vi "VI_PC.vi"() -> ()   [LabVIEW 2018]
uses:
  <vilib>/Utility/inputDevices.llb/joystickAcquire.vi
  <vilib>/Utility/inputDevices.llb/closeJoystick.vi
panel:
  out "direction info":T1
  out "button info":T2
  out "axis info":T3
  in  "stop":bool
  out "error out":errorcluster
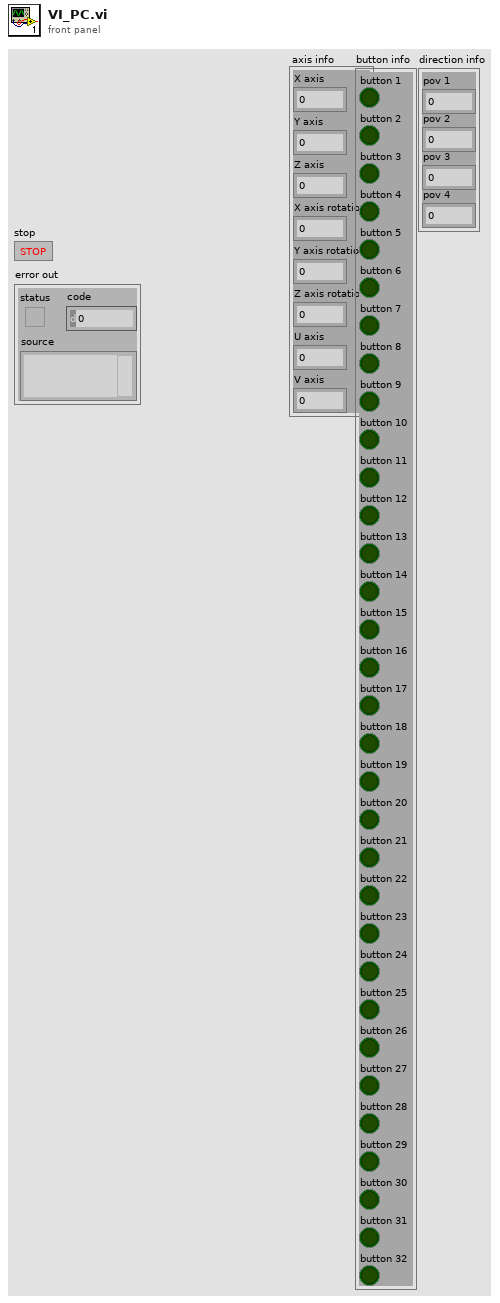
[diagram p1: front panel]
types:
  T1 = cluster{"pov 1":i32, "pov 2":i32, "pov 3":i32, "pov 4":i32}
  T2 = cluster{"button 1":bool, "button 2":bool, "button 3":bool, "button 4":bool, "button 5":bool, "button 6":bool, "button 7":bool, "button 8":bool, "button 9":bool, "button 10":bool, "button 11":bool, "button 12":bool, "button 13":bool, "button 14":bool, "button 15":bool, "button 16":bool, "button 17":bool, "button 18":bool, "button 19":bool, "button 20":bool, "button 21":bool, "button 22":bool, "button 23":bool, "button 24":bool, "button 25":bool, "button 26":bool, "button 27":bool, "button 28":bool, "button 29":bool, "button 30":bool, "button 31":bool, "button 32":bool}
  T3 = cluster{"X axis":i32, "Y axis":i32, "Z axis":i32, "X axis rotation":i32, "Y axis rotation":i32, "Z axis rotation":i32, "U axis":i32, "V axis":i32}
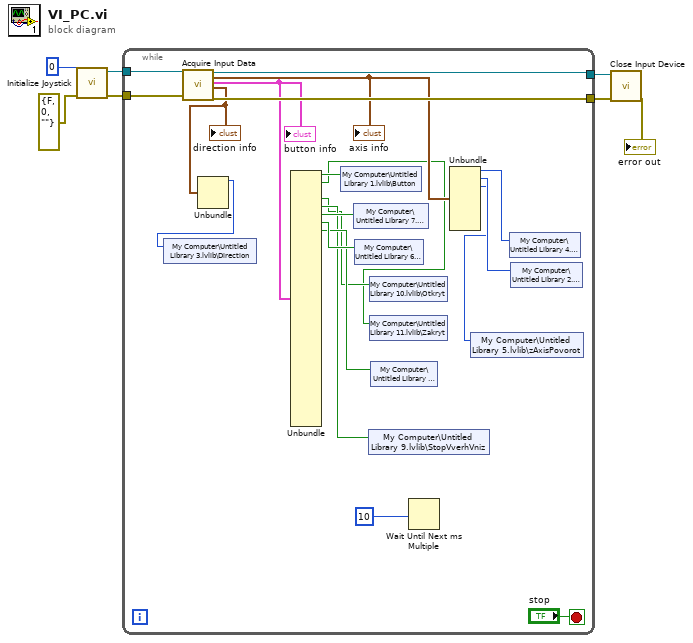
[diagram p0: block diagram]
diagram:
  n1 = call <vilib>:"Initialize Joystick.vi"("error in (no error)"=errorcluster {"status"=FALSE, "code"=0, "source"=""}, "device index"=0) -> ("error out"=w7:errorcluster, "device ID"=w6:refnum<k1>)  [unwired: 8 in]
  n2 = while {
    tunnel: w7 -> [w27]
    tunnel: w6 -> [w26]
    tunnel: [w25] -> w3
    tunnel: [w24] -> w2
    stop <- "stop" stop-if-true
    n3 = call-poly <vilib>:"Acquire Input Data.vi"("device ID"=w26, "error in (no error)"=w27) -> ("device ID"=w24:refnum<k1>, "axis info"=w19:T3, "button info"=w22:T2, "direction info"=w20:T1, "error out"=w25:errorcluster)  [unwired: 13 in]
    "axis info" <- w19
    "button info" <- w22
    "direction info" <- w20
    n4 = Unbundle(w20) -> ("pov 1"=w18:i32)  [unwired: 3 out]
    n5 = shared-variable "My Computer\\Untitled Library 3.lvlib\\Direction"(w18) -> ()  [unwired: 1 in, 1 out]
    n6 = Unbundle(w22) -> ("button 1"=w21:bool, "button 2"=w8:bool, "button 4"=w9:bool, "button 5"=w10:bool, "button 6"=w12:bool, "button 7"=w13:bool, "button 8"=w11:bool)  [unwired: 25 out]
    n7 = shared-variable "My Computer\\Untitled Library 1.lvlib\\Button"(w21) -> ()  [unwired: 1 in, 1 out]
    n8 = shared-variable "My Computer\\Untitled Library 7.lvlib\\Vverh"(w12) -> ()  [unwired: 1 in, 1 out]
    n9 = shared-variable "My Computer\\Untitled Library 6.lvlib\\Stop"(w13) -> ()  [unwired: 1 in, 1 out]
    n10 = shared-variable "My Computer\\Untitled Library 9.lvlib\\StopVverhVniz"(w10) -> ()  [unwired: 1 in, 1 out]
    n11 = shared-variable "My Computer\\Untitled Library 10.lvlib\\Otkryt"(w9) -> ()  [unwired: 1 in, 1 out]
    n12 = shared-variable "My Computer\\Untitled Library 11.lvlib\\Zakryt"(w8) -> ()  [unwired: 1 in, 1 out]
    n13 = shared-variable "My Computer\\Untitled Library 8.lvlib\\Vniz"(w11) -> ()  [unwired: 1 in, 1 out]
    n14 = Wait Until Next ms Multiple(millisecond multiple=10) -> ()  [unwired: 1 out]
    n15 = Unbundle(w19) -> ("X axis"=w15:i32, "Y axis"=w17:i32, "Z axis"=w14:i32)  [unwired: 5 out]
    n16 = shared-variable "My Computer\\Untitled Library 5.lvlib\\zAxisPovorot"(w14) -> ()  [unwired: 1 in, 1 out]
    n17 = shared-variable "My Computer\\Untitled Library 4.lvlib\\xAxis"(w15) -> ()  [unwired: 1 in, 1 out]
    n18 = shared-variable "My Computer\\Untitled Library 2.lvlib\\yAxis"(w17) -> ()  [unwired: 1 in, 1 out]
  }
  n19 = call-poly <vilib>:"Close Input Device.vi"("error in (no error)"=w3, "device ID"=w2) -> ("error out"=→"error out":errorcluster)  [unwired: 8 in]
